vi "Get Instrument Address.vi"(8 "error in (no error)":errorcluster, 11 "Instrument Properties in":refnum<class "Instrument Properties.lvclass">) -> (0 "error out":errorcluster, 2 "Instrument Address":string, 3 "Instrument Properties out":refnum<class "Instrument Properties.lvclass">)   [LabVIEW 2015, in "Instrument.lvlib" / "Instrument Properties.lvclass"]
uses:
  Instrument Properties.lvclass
  Instrument Properties.lvclass/Instrument Properties.ctl
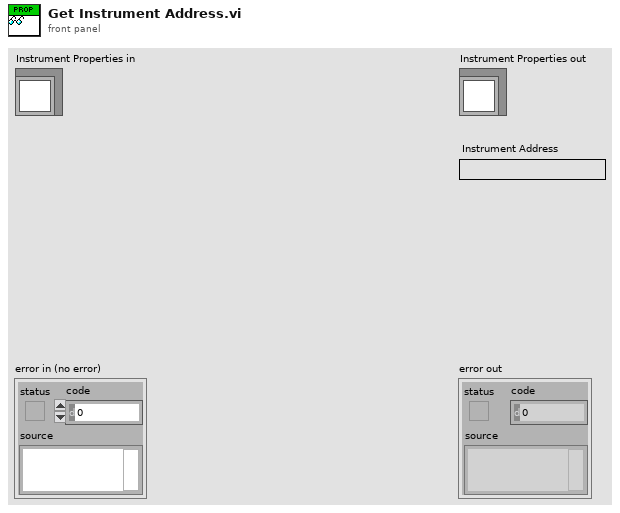
[diagram p1: front panel]
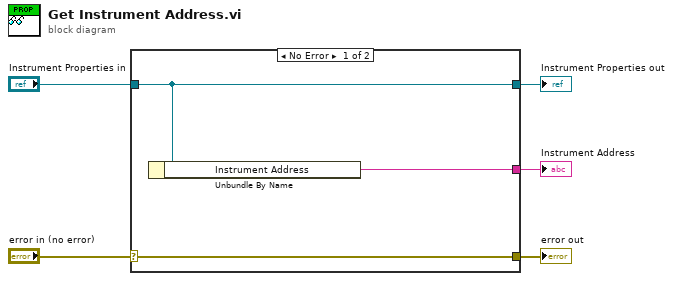
[diagram p0: block diagram]
diagram:
  n1 = case shown="No Error" "error in (no error)" {
    selector: "error in (no error)" -> [w8 w9]
    tunnel: [w8 w9] -> w4
    tunnel: [w7 w10] -> w2
    tunnel: "Instrument Properties in" -> [w7 w10]
    tunnel: [w6 _] -> w1
    frame No Error {
      n2 = Unbundle By Name(w7) -> ("Instrument Address"=w6:string)
    }
    frame Error {
    }
  }
  "error out" <- w4
  "Instrument Properties out" <- w2
  "Instrument Address" <- w1
